vi "Read N Channels.vi"(8 "error in":errorcluster, 10 "Channels":variant, 11 "DI DAQmx Cont CFG in":refnum<class "DI DAQmx Cont CFG.lvclass">) -> (0 "error out":errorcluster, 2 "Readings":variant, 3 "DI DAQmx Cont CFG out":refnum<class "DI DAQmx Cont CFG.lvclass">)   [LabVIEW 2024, in "DI DAQmx Cont CFG.lvclass"]
uses:
  DI DAQmx Cont CFG.lvclass
  DI DAQmx Cont CFG.lvclass/DI DAQmx Cont CFG.ctl
  DAQmx Base CFG/DAQmx Base CFG.lvclass
  <vilib>/DAQmx/read.llb/DAQmx Read (Digital 1D Wfm NChan NSamp).vi
  Buffers/Buffer Lossless Digital/Buffer Lossless Digital.lvclass
  D:/git/HAL/HAL/Devices/DAQmx/DAQmx Base CFG/DAQmx Base CFG.lvclass
  D:/git/HAL/HAL/Configurations/CFG Base/CFG Base.lvclass
  D:/git/HAL/HAL/Devices/DAQmx/DIO/DI DAQmx Cont CFG/DI DAQmx Cont CFG.lvclass
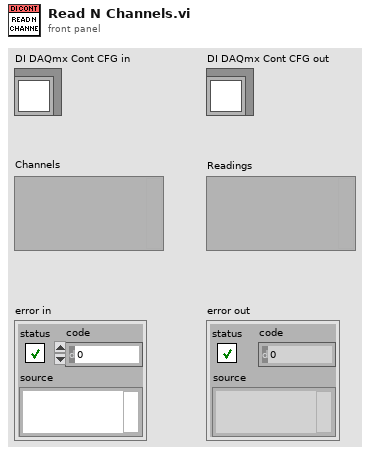
[diagram p1: front panel]
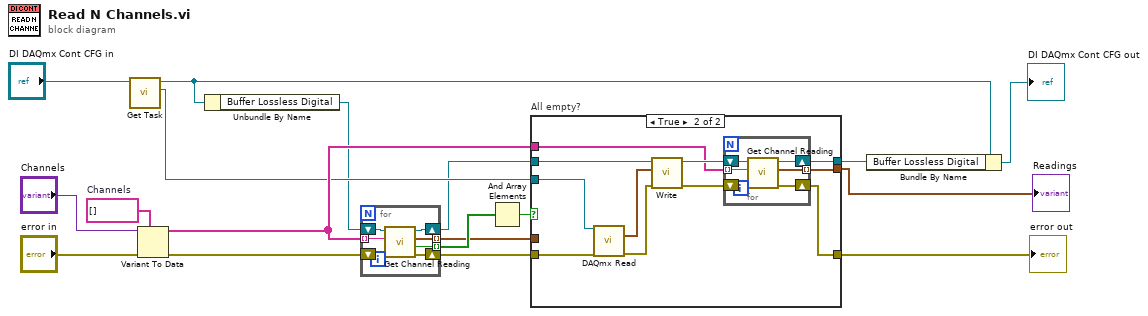
[diagram p0: block diagram]
diagram:
  w11 = string[] []  # Channels
  n1 = call "Get Task.vi"("DAQmx Base CFG in"="DI DAQmx Cont CFG in") -> ("Task"=w15:refnum<k21>, "DAQmx Base CFG out"=w18:refnum<class "DI DAQmx Cont CFG.lvclass">)  [unwired: 9 in]
  n2 = Variant To Data(error in="error in", type=w11, Variant="Channels") -> (data=w17:string[], error out=w16:errorcluster)
  n3 = Unbundle By Name(w18) -> ("Buffer Lossless Digital"=w7:refnum<class "Buffer Lossless Digital.lvclass">)
  n4 = for {
    tunnel: [w22] -> w3 mode=indexing
    shift-right: [w24] -> w8
    shift-left: w16 -> [w25]
    shift-right: [w21] -> w6
    shift-left: w7 -> [w23]
    tunnel: w17 -> [w20] mode=indexing
    tunnel: [w19] -> w5 mode=indexing
    n5 = call "Get Channel Reading.vi"("error in"=w25, "Channel"=w20, "Buffer Lossless Bin in"=w23) -> ("error out"=w24:errorcluster, "empty?"=w19:bool, "Reading"=w22:digitalwaveform, "Buffer Lossless Bin out"=w21:refnum<class "Buffer Lossless Digital.lvclass">)  [unwired: 5 in]
  }
  n6 = And Array Elements(Boolean array=w5) -> (logical AND=w4:bool)
  n7 = case "All empty?" shown="True" w4 {
    tunnel: [w26 w30] -> w2
    tunnel: [w27 w33] -> w9
    tunnel: [w28 w29] -> w1
    tunnel: w6 -> [w27 w39]
    tunnel: w17 -> [_ w31]
    tunnel: w8 -> [w26 w38]
    tunnel: w15 -> [_ w37]
    tunnel: w3 -> [w28 _]
    frame False {
    }
    frame True {
      n8 = call-poly <vilib>:"DAQmx Read.vi"("task/channels in"=w37, "error in"=w38) -> ("data"=w35:digitalwaveform[], "error out"=w36:errorcluster)  [unwired: 11 in, 1 out]
      n9 = call "Write.vi"("error in"=w36, "Readings"=w35, "Buffer Lossless Digital in"=w39) -> ("error out"=w32:errorcluster, "Buffer Lossless Digital out"=w34:refnum<class "Buffer Lossless Digital.lvclass">)  [unwired: 7 in]
      n10 = for {
        shift-right: [w44] -> w33
        shift-left: w34 -> [w45]
        shift-right: [w40] -> w30
        shift-left: w32 -> [w41]
        tunnel: w31 -> [w43] mode=indexing
        tunnel: [w42] -> w29 mode=indexing
        n11 = call "Get Channel Reading.vi"("error in"=w41, "Channel"=w43, "Buffer Lossless Bin in"=w45) -> ("error out"=w40:errorcluster, "Reading"=w42:digitalwaveform, "Buffer Lossless Bin out"=w44:refnum<class "Buffer Lossless Digital.lvclass">)  [unwired: 5 in, 1 out]
      }
    }
  }
  "error out" <- w2
  "Readings" <- w1
  n12 = Bundle By Name(cluster=w18, "Buffer Lossless Digital"=w9) -> (→"DI DAQmx Cont CFG out":refnum<class "DI DAQmx Cont CFG.lvclass">)
